vi "Main.vi"() -> ()   [LabVIEW 2014]
doc: "This Continuous Measurement sample project is based on the Queued Message Handler template.\n\nThe Event Handling Loop generates messages based on user interface actions.\n\nThe Message Handling Loop processes messages generated by the Event Handling Loop, or by other messages. There are also Acquisition and Logging message handling loop subVIs, and a chart updating loop."
uses:
  Settings/Settings.ctl
  Acquisition/Hardware Configuration.ctl
  Logging/Logging Configuration.ctl
  controls/UI Data.ctl
  controls/UI State.ctl
  support/Message Queue/Enqueue Message (Single).vi
  <vilib>/Utility/error.llb/Error Cluster From Error Code.vi
  <vilib>/ErrorRing/Error Ring.xnode
  Acquisition/Acquisition.lvlib
  Logging/Logging.lvlib
  Settings/Settings.lvlib
  support/User Event - Stop/User Event - Stop.lvlib
  support/Message Queue/Message Queue.lvlib
panel:
  out "Data":waveform(dbl)[](graph)
  in  "UserMetaData":T1 {"Amplifier Model" items=["Select a Model", "AM 1700", "BMA 200"]}
  in  "Settings":bool
  in  "Start":bool
  in  "Stop":bool
  out "Status":string
  in  "Exit":bool
  # "Direct-To-Disk Long Term EOD Recording Software (TDMS Output) (1.0)"
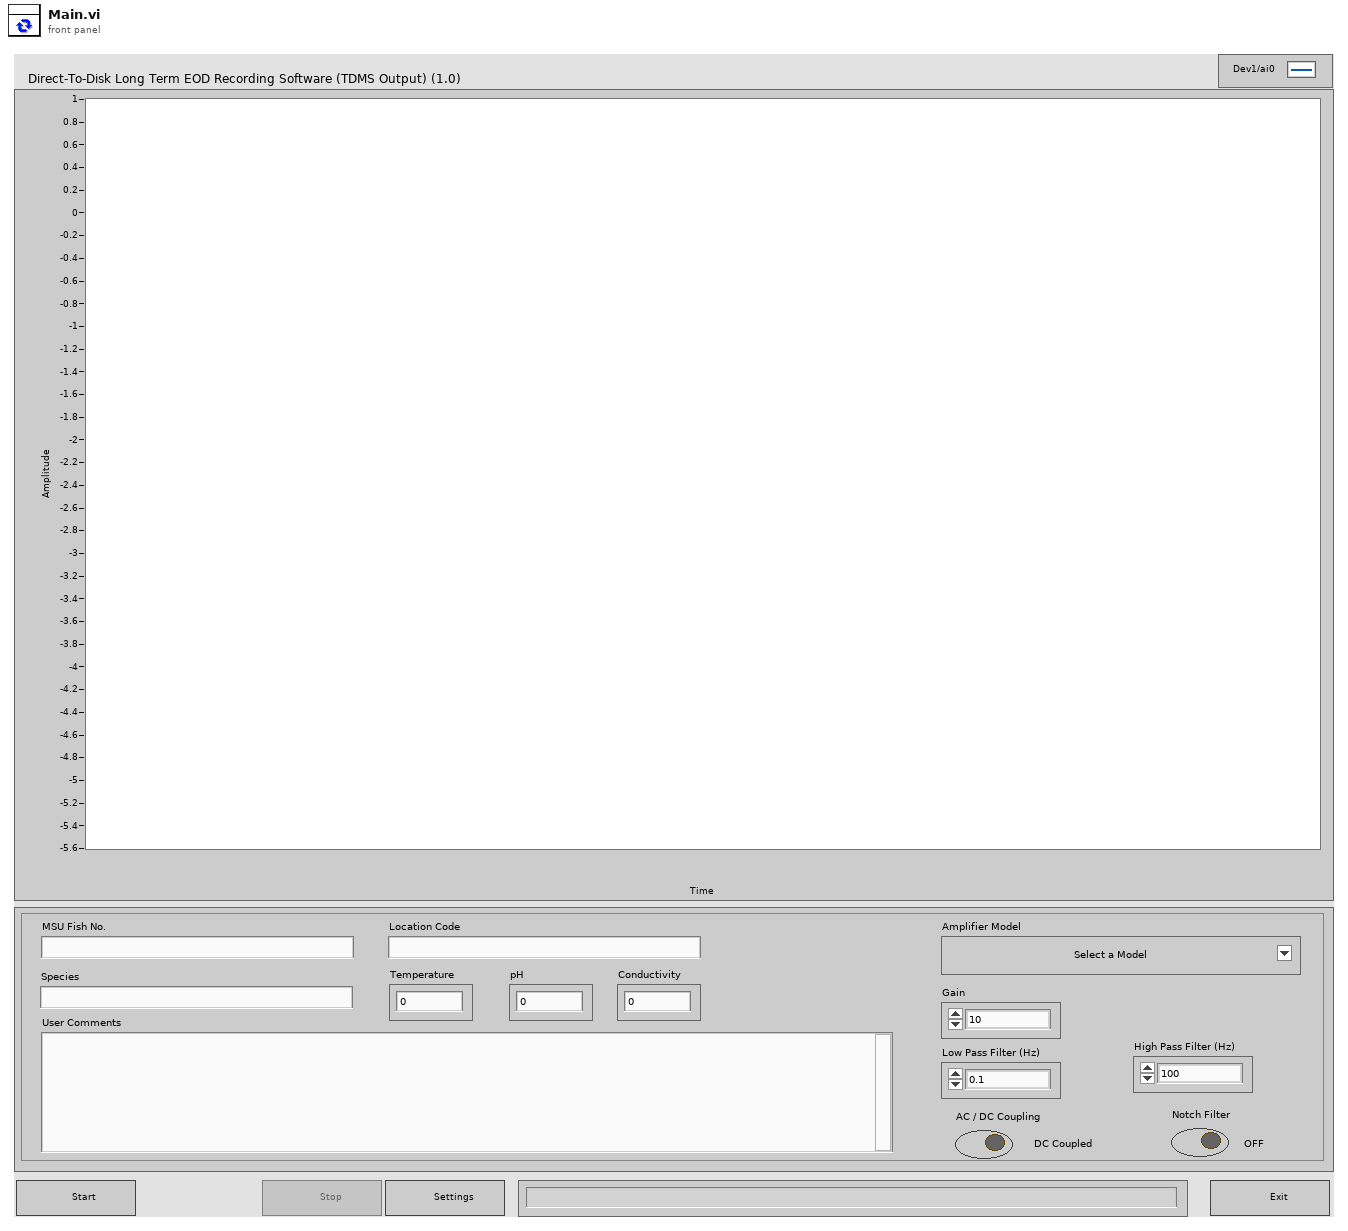
[diagram p1: front panel]
types:
  T1 = cluster{"MSU Fish No.":string, "Location Code":string, "Species":string, "Temperature":dbl, "pH":dbl, "Conductivity":dbl, "User Comments":string, "Amplifier Model":u16, "Gain":enum16{"10", "20", "50", "100", "200", "500", "1000", "2k", "5k", "10k", "20k", "50k"}, "Low Pass Filter (Hz)":enum16{"0.1", "1", "3", "10", "30", "100", "300"}, "High Pass Filter (Hz)":enum16{"100", "500", "1000", "3000", "5000", "10,000", "20,000", "30,000", "50,000"}, "AC / DC Coupling":bool, "Notch Filter":bool}
  T2 = typedef "UI State.ctl" = enum16{"Idle", "Acquiring and Logging", "Waiting for Exit", "Waiting for Exit (Acq Stopped)", "Waiting for Exit (Log Stopped)", "Waiting for Stop", "Waiting for Stop (Acq Stopped)", "Waiting for Stop (Log Stopped)"}
  T3 = typedef "UI Data.ctl" = cluster{"Start Ref":refnum<vi>, "Trigger Ref":refnum<vi>, "Stop Ref":refnum<vi>, "Settings Ref":refnum<vi>, "Status Ref":refnum<vi>, "Exit Ref":refnum<vi>, "Data Ref":refnum<vi>}
  T4 = typedef "Settings.lvlib/Settings.ctl" = cluster{"Hardware Configuration":T5, "Logging Configuration":T6}
  T5 = typedef "Acquisition.lvlib/Hardware Configuration.ctl" = cluster{"DAQmx Channel":tag, "Max Input":dbl, "Min Input":dbl, "Sample Rate":dbl, "DAQmx Task":refnum<k21>}
  T6 = typedef "Logging.lvlib/Logging Configuration.ctl" = cluster{"Log File Base Path":path, "TDMS File Reference":refnum<k34>, "Samples to Save":u32, "Trigger - Time":u32, "Trigger - Threshold":dbl, "Trigger - Channel":u32, "Enable Time Trigger":bool, "Enable Threshold Trigger":bool, "Always Log":bool}
  T7 = typedef "Message Queue.lvlib/All Message Queues.ctl" = cluster{"UI":refnum<queue>, "Acquisition":refnum<queue>, "Logging":refnum<queue>}
  T8 = enum8{"Enabled", "Disabled", "Disabled and Grayed Out"}
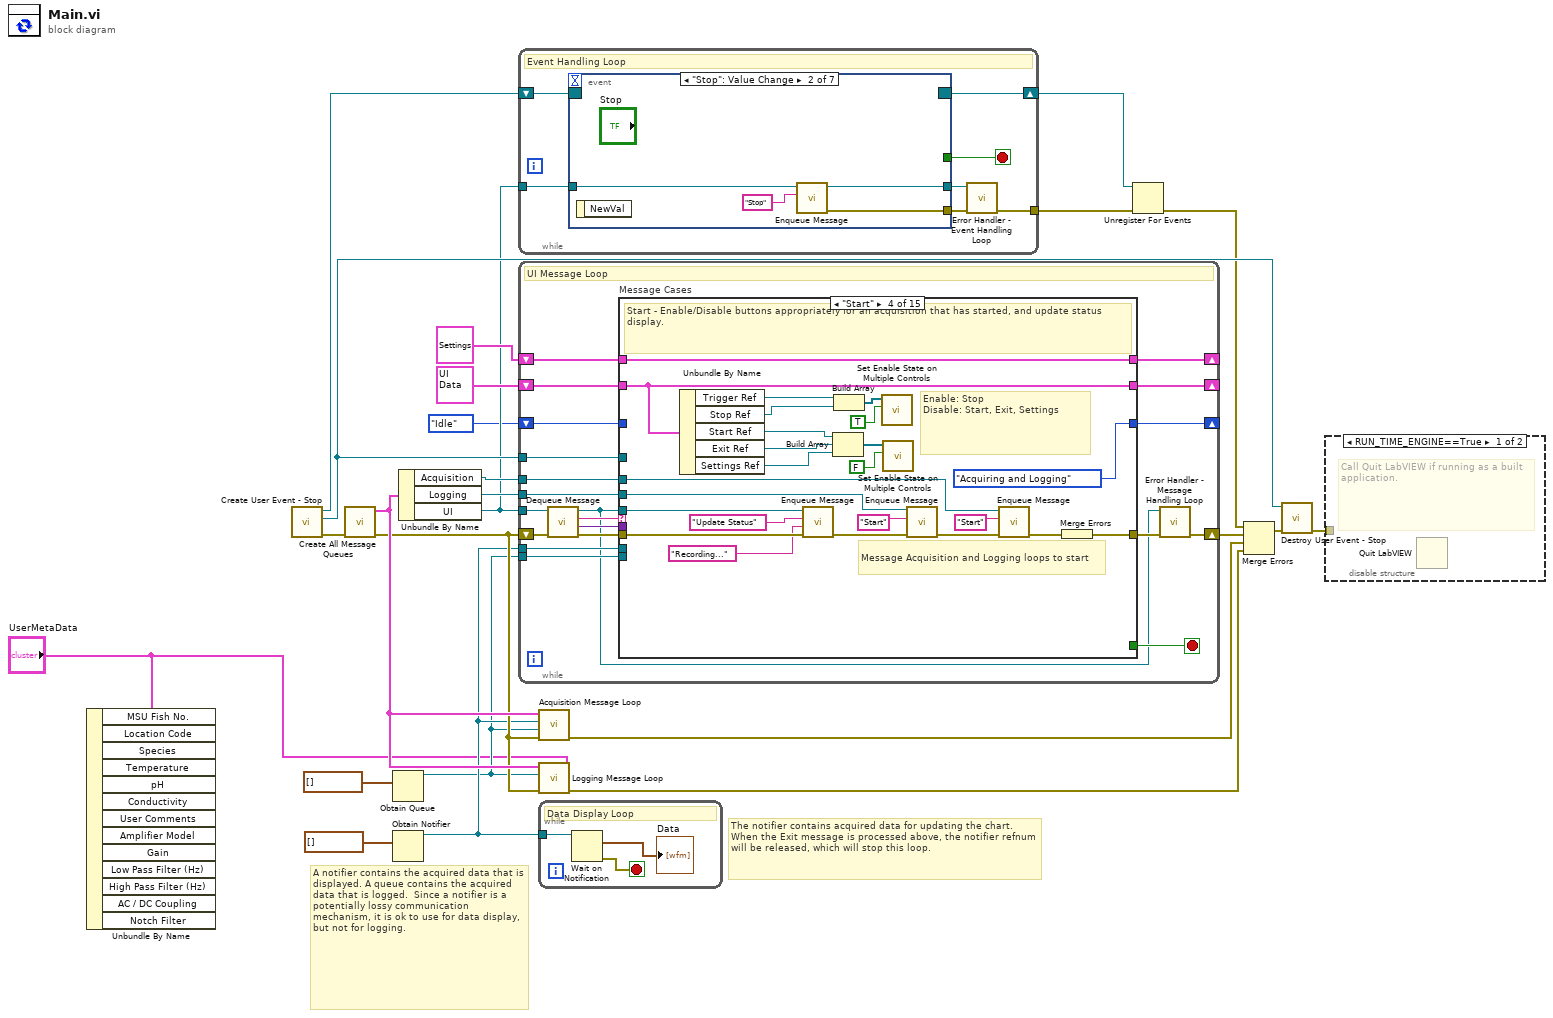
[diagram p0: block diagram]
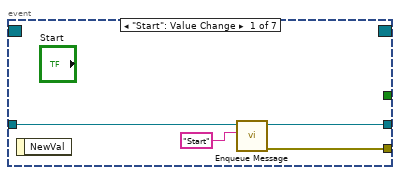
[diagram p3: hidden frame]
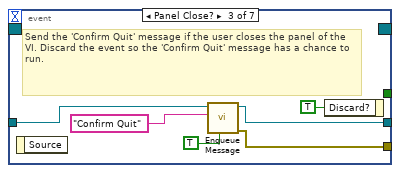
[diagram p4: hidden frame]
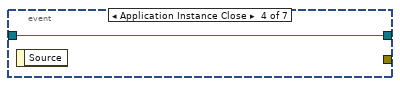
[diagram p5: hidden frame]
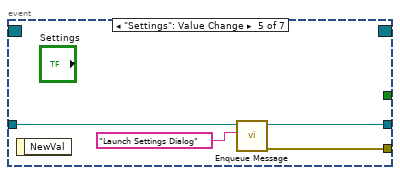
[diagram p6: hidden frame]
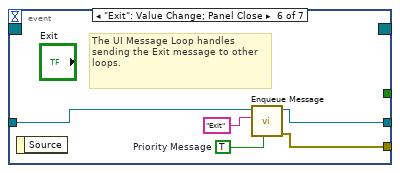
[diagram p7: hidden frame]
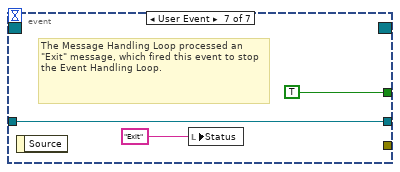
[diagram p8: hidden frame]
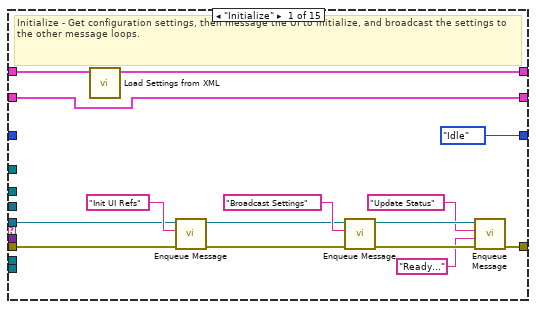
[diagram p9: hidden frame]
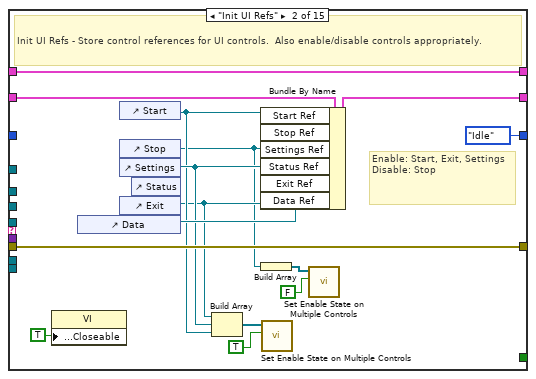
[diagram p10: hidden frame]
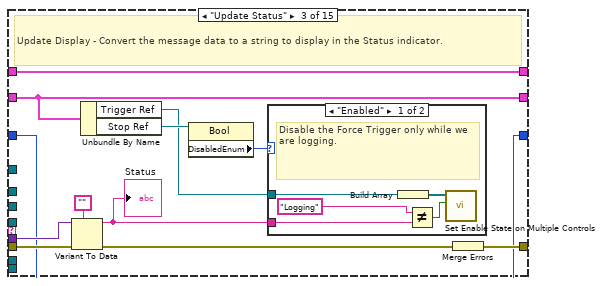
[diagram p11: hidden frame]
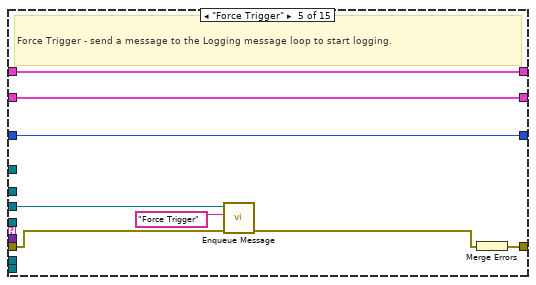
[diagram p13: hidden frame]
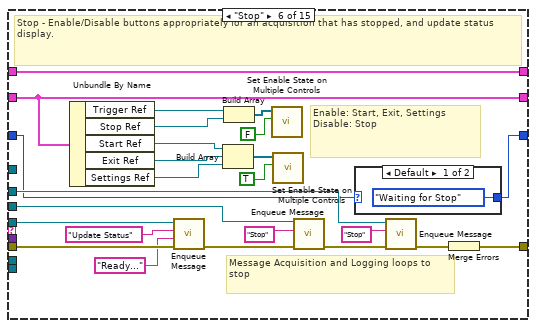
[diagram p14: hidden frame]
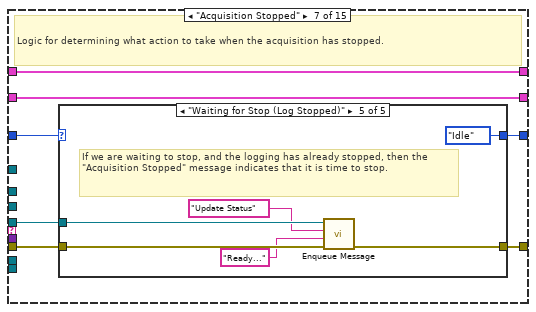
[diagram p16: hidden frame]
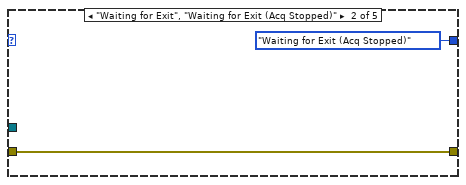
[diagram p18: hidden frame]
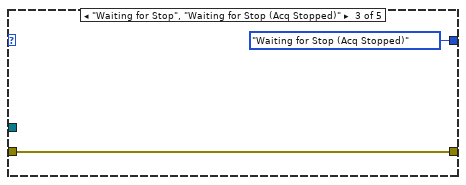
[diagram p19: hidden frame]
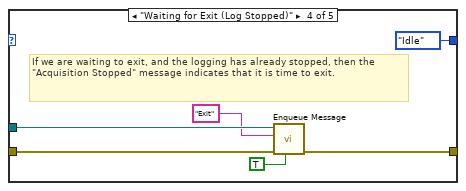
[diagram p20: hidden frame]
diagram:
  # "A notifier contains the acquired data that is displayed. A queue contains the acquired data that is logged.  Since a notifier is a potentially lossy communication mechanism, it is ok to use for data display, but not for logging."
  # "The notifier contains acquired data for updating the chart. When the Exit message is processed above, the notifier refnum will be released, which will stop this loop."
  n1 = Unbundle By Name("UserMetaData") -> ()  [unwired: 13 out]
  n2 = call "Create User Event - Stop.vi"() -> ("error out"=w18:errorcluster, "User Event - Stop"=w20:refnum<user-event>, "Stop Event Registration Refnum"=w21:refnum<event-registration>)  [unwired: 9 in]
  n3 = call "Create All Message Queues.vi"("error in (no error)"=w18) -> ("error out"=w15:errorcluster, "Message Queues out"=w17:T7)  [unwired: 9 in]
  n4 = Obtain Queue(element data type=waveform(dbl)[] []) -> (queue out=w4:refnum<queue>)  [unwired: 4 in, 2 out]
  n5 = Obtain Notifier(notification data type=waveform(dbl)[] []) -> (notifier out=w6:refnum<notifier>)  [unwired: 3 in, 2 out]
  n6 = Unbundle By Name(w17) -> ("Acquisition"=w10:refnum<queue>, "Logging"=w9:refnum<queue>, "UI"=w8:refnum<queue>)
  n7 = while {
    tunnel: w8 -> [w30]
    tunnel: [w25] -> w23
    shift-right: [w29] -> w12
    shift-left: w21 -> [w31]
    stop <- w28 stop-if-true
    # "Event Handling Loop"
    n8 = event shown="[1] \"Stop\": Value Change" {
      selector: w31 -> [_ _ _ _ _ _ _]
      dyn-events: [_ _ _ _ _ _ _] -> w29
      timeout: _ -> [_ _ _ _ _ _ _]
      tunnel: [_ _ _ _ _ _ TRUE ("Discard?")] -> w28
      tunnel: w30 -> [w33 w38 w45 w46 w48 w52 w56]
      tunnel: [w35 w37 w40 _ w50 w55 _] -> w26
      tunnel: [w32 w36 w41 w46 w47 w51 w56] -> w27
      event "Start": Value Change {
        n9 = event-data() -> ()  [unwired: 1 in, 1 out]
        n10 = call-poly "Enqueue Message.vi"("Message"="Start", "Message Queue"=w33) -> ("error out"=w35:errorcluster, "dup Message Queue"=w32:refnum<queue>)  [unwired: 8 in]
      }
      event "Stop": Value Change {
        n11 = event-data() -> ()  [unwired: 1 in, 1 out]
        n12 = call-poly "Enqueue Message.vi"("Message"="Stop", "Message Queue"=w38) -> ("error out"=w37:errorcluster, "dup Message Queue"=w36:refnum<queue>)  [unwired: 8 in]
      }
      event Panel Close? {
        # "Send the 'Confirm Quit' message if the user closes the panel of the VI. Discard the event so the 'Confirm Quit' message has a chance to run."
        n13 = event-data() -> ()  [unwired: 1 in, 1 out]
        n14 = call-poly "Enqueue Message.vi"("Priority Message? (F)"=TRUE, "Message"="Confirm Quit", "Message Queue"=w45) -> ("error out"=w40:errorcluster, "dup Message Queue"=w41:refnum<queue>)  [unwired: 7 in]
        n15 = event-data("Discard?"=TRUE) -> ()  [unwired: 1 in, 1 out]
      }
      event Application Instance Close {
        n16 = event-data() -> ()  [unwired: 1 in, 1 out]
      }
      event "Settings": Value Change {
        n17 = event-data() -> ()  [unwired: 1 in, 1 out]
        n18 = call-poly "Enqueue Message.vi"("Message"="Launch Settings Dialog", "Message Queue"=w48) -> ("error out"=w50:errorcluster, "dup Message Queue"=w47:refnum<queue>)  [unwired: 8 in]
      }
      event "Exit": Value Change; Panel Close {
        w53 = TRUE  # Priority Message
        # "The UI Message Loop handles sending the Exit message to other loops."
        n19 = event-data() -> ()  [unwired: 1 in, 1 out]
        n20 = call-poly "Enqueue Message.vi"("Priority Message? (F)"=w53, "Message"="Exit", "Message Queue"=w52) -> ("error out"=w55:errorcluster, "dup Message Queue"=w51:refnum<queue>)  [unwired: 7 in]
      }
      event User Event {
        # "The Message Handling Loop processed an \"Exit\" message, which fired this event to stop the Event Handling Loop."
        n21 = event-data() -> ()  [unwired: 1 in, 1 out]
        n22 = local write "Status"("Exit" ("Exit String")) -> ()
      }
    }
    n23 = call "Error Handler - Event Handling Loop.vi"("error in (no error)"=w26, "Message Queue"=w27) -> ("dup error in"=w25:errorcluster)  [unwired: 8 in, 1 out]
  }
  n24 = while {
    tunnel: w8 -> [w72]
    tunnel: w20 -> [w77]
    shift-right: [w62] -> w24
    shift-left: w15 -> [w76]
    shift-right: [w71] -> _
    shift-left: T4 {"Hardware Configuration"={"DAQmx Channel"="", "Max Input"=0.0, "Min Input"=0.0, "Sample Rate"=0.0, "DAQmx Task"=""}, "Logging Configuration"={"Log File Base Path"=path "", "TDMS File Reference"=refnum, "Samples to Save"=0, "Trigger - Time"=0, "Trigger - Threshold"=0.0, "Trigger - Channel"=0, "Enable Time Trigger"=FALSE, "Enable Threshold Trigger"=FALSE, "Always Log"=FALSE}} ("Settings") -> [w70]
    shift-right: [w68] -> _
    shift-left: T3 {"Start Ref"=refnum, "Trigger Ref"=refnum, "Stop Ref"=refnum, "Settings Ref"=refnum, "Status Ref"=refnum, "Exit Ref"=refnum, "Data Ref"=refnum} ("Measurement UI Controls") -> [w69]
    tunnel: w10 -> [w67]
    tunnel: w9 -> [w66]
    tunnel: w6 -> [w65]
    tunnel: w4 -> [w64]
    shift-right: [w59] -> _
    shift-left: UI_State."Idle" ("UI State") -> [w60]
    stop <- w78 stop-if-true
    # "UI Message Loop"
    n25 = call "Dequeue Message.vi"("error in (no error)"=w76, "Message Queue"=w72) -> ("error out"=w75:errorcluster, "Message Data"=w73:variant, "Message"=w74:string, "dup Message Queue"=w61:refnum<queue>)  [unwired: 6 in]
    n26 = case "Message Cases" shown="\"Start\"" w74 {
      selector: w74 -> [_ _ _ _ _ _ _ _ _ _ _ _ _ _ w328]
      tunnel: w61 -> [w83 _ _ w149 _ w182 w186 w211 _ w253 w268 w278 w311 _ _]
      tunnel: w75 -> [w82 w109 w120 w148 w155 w181 w188 w213 w241 w255 w272 w277 w319 w326 _]
      tunnel: [w89 w109 w121 w150 w158 w183 w187 w212 w247 w250 w263 w276 w320 w325 w329] -> w63
      tunnel: [_ _ _ _ _ _ _ _ _ _ _ _ TRUE _ _] -> w78
      tunnel: w73 -> [_ _ w119 _ _ _ _ _ _ _ w271 _ _ _ _]
      tunnel: w77 -> [_ _ _ _ _ _ _ _ _ _ _ _ w318 _ _]
      tunnel: [w92 w108 w116 w147 w157 w180 w192 w217 w245 w252 w274 w281 w316 w324 w331] -> w71
      tunnel: w70 -> [w93 w108 w116 w147 w157 w180 w192 w217 w245 w256 w274 w281 w316 w324 w331]
      tunnel: w69 -> [w85 w107 w115 w144 w156 w177 w191 w216 w239 w249 w273 w280 w314 w323 w330]
      tunnel: [w85 w106 w115 w144 w156 w177 w191 w216 w239 w249 w273 w280 w314 w323 w330] -> w68
      tunnel: w67 -> [_ _ _ w131 _ w164 _ _ w238 _ _ _ w313 _ _]
      tunnel: w66 -> [_ _ _ w134 w152 w167 _ _ w237 _ _ _ w312 _ _]
      tunnel: w65 -> [_ _ _ _ _ _ _ _ _ _ _ _ w310 _ _]
      tunnel: w64 -> [_ _ _ _ _ _ _ _ _ _ _ _ w306 _ _]
      tunnel: w60 -> [_ _ w110 _ w151 w160 w190 w215 w236 w248 w262 w279 _ w322 w327]
      tunnel: [UI_State."Idle" ("UI State") UI_State."Idle" ("UI State") w110 UI_State."Acquiring and Logging" ("UI State") w151 w159 w189 w214 w236 w248 w262 w275 UI_State."Idle" ("UI State") w322 w327] -> w59
      frame "Initialize" {
        # "Initialize - Get configuration settings, then message the UI to initialize, and broadcast the settings to the other message loops."
        n27 = call "Load Settings from XML.vi"("Settings in"=w93) -> ("Settings out"=w92:T4)  [unwired: 9 in, 1 out]
        n28 = call-poly "Enqueue Message.vi"("error in (no error)"=w82, "Message"="Init UI Refs", "Message Queue"=w83) -> ("error out"=w80:errorcluster, "dup Message Queue"=w81:refnum<queue>)  [unwired: 7 in]
        n29 = call-poly "Enqueue Message.vi"("error in (no error)"=w80, "Message"="Broadcast Settings", "Message Queue"=w81) -> ("error out"=w91:errorcluster, "dup Message Queue"=w90:refnum<queue>)  [unwired: 7 in]
        n30 = call-poly "Enqueue Message.vi"("error in (no error)"=w91, "Message Data"="Ready..." ("Ready..."), "Message"="Update Status", "Message Queue"=w90) -> ("error out"=w89:errorcluster)  [unwired: 6 in, 1 out]
      }
      frame "Init UI Refs" {
        # "Enable: Start, Exit, Settings\nDisable: Stop"
        # "Init UI Refs - Store control references for UI controls.  Also enable/disable controls appropriately."
        n31 = property class="VI"("Front Panel.Closeable"=TRUE ("Front Panel Window:Closeable")) -> ()  [unwired: 2 in, 2 out]
        n32 = control-ref of="Data"() -> (w102:refnum<vi>)
        n33 = control-ref of="Start"() -> (w101:refnum<vi>)
        n34 = control-ref of="Stop"() -> (w96:refnum<vi>)
        n35 = control-ref of="Settings"() -> (w98:refnum<vi>)
        n36 = control-ref of="Exit"() -> (w97:refnum<vi>)
        n37 = control-ref of="Status"() -> (w103:refnum<vi>)
        n38 = Build Array(w97, w98, w101) -> (w100:refnum<vi>[])
        n39 = Bundle By Name(cluster=w107, "Start Ref"=w101, "Stop Ref"=w96, "Settings Ref"=w98, "Status Ref"=w103, "Exit Ref"=w97, "Data Ref"=w102) -> (w106:T3)
        n40 = Build Array(w96) -> (w95:refnum<vi>[])
        n41 = call "Set Enable State on Multiple Controls.vi"("Enable?"=TRUE, "Controls"=w100) -> ()  [unwired: 10 in]
        n42 = call "Set Enable State on Multiple Controls.vi"("Enable?"=FALSE, "Controls"=w95) -> ()  [unwired: 10 in]
      }
      frame "Update Status" {
        # "Update Display - Convert the message data to a string to display in the Status indicator."
        n43 = Variant To Data(error in=w120, type="", Variant=w119) -> (data=w112:string, error out=w117:errorcluster)
        "Status" <- w112
        n44 = Unbundle By Name(w115) -> ("Trigger Ref"=w111:refnum<vi>, "Stop Ref"=w114:refnum<vi>)
        n45 = property class="Bool"(reference=w114) -> ("DisabledEnum"=w113:T8)  [unwired: 1 in, 2 out]
        n46 = case shown="\"Enabled\"" w113 {
          tunnel: w112 -> [w124 _]
          tunnel: w111 -> [w125 _]
          frame "Enabled" {
            # "Disable the Force Trigger only while we are logging."
            n47 = Build Array(w125) -> (w126:refnum<vi>[])
            n48 = Not Equal?(x="Logging" ("Logging"), y=w124) -> (x != y?=w122:bool)
            n49 = call "Set Enable State on Multiple Controls.vi"("Enable?"=w122, "Controls"=w126) -> ()  [unwired: 10 in]
          }
          frame "Disabled", Default {
          }
        }
        n50 = Merge Errors(w117) -> (w121:errorcluster)
      }
      frame "Start" {
        # "Message Acquisition and Logging loops to start"
        # "Enable: Stop\nDisable: Start, Exit, Settings"
        # "Start - Enable/Disable buttons appropriately for an acquisition that has started, and update status display."
        n51 = Unbundle By Name(w144) -> ("Trigger Ref"=w128:refnum<vi>, "Stop Ref"=w129:refnum<vi>, "Start Ref"=w139:refnum<vi>, "Exit Ref"=w138:refnum<vi>, "Settings Ref"=w137:refnum<vi>)
        n52 = call-poly "Enqueue Message.vi"("error in (no error)"=w148, "Message Data"="Recording..." ("Waiting for trigger"), "Message"="Update Status", "Message Queue"=w149) -> ("error out"=w136:errorcluster)  [unwired: 6 in, 1 out]
        n53 = Build Array(w139, w138, w137) -> (w142:refnum<vi>[])
        n54 = Build Array(w128, w129) -> (w141:refnum<vi>[])
        n55 = call "Set Enable State on Multiple Controls.vi"("Enable?"=TRUE, "Controls"=w141) -> ()  [unwired: 10 in]
        n56 = call "Set Enable State on Multiple Controls.vi"("Enable?"=FALSE, "Controls"=w142) -> ()  [unwired: 10 in]
        n57 = call-poly "Enqueue Message.vi"("error in (no error)"=w136, "Message"="Start", "Message Queue"=w134) -> ("error out"=w133:errorcluster)  [unwired: 7 in, 1 out]
        n58 = call-poly "Enqueue Message.vi"("error in (no error)"=w133, "Message"="Start", "Message Queue"=w131) -> ("error out"=w132:errorcluster)  [unwired: 7 in, 1 out]
        n59 = Merge Errors(w132) -> (w150:errorcluster)
      }
      frame "Force Trigger" {
        # "Force Trigger - send a message to the Logging message loop to start logging."
        n60 = call-poly "Enqueue Message.vi"("error in (no error)"=w155, "Message"="Force Trigger", "Message Queue"=w152) -> ("error out"=w154:errorcluster)  [unwired: 7 in, 1 out]
        n61 = Merge Errors(w154) -> (w158:errorcluster)
      }
      frame "Stop" {
        # "Message Acquisition and Logging loops to stop"
        # "Enable: Start, Exit, Settings\nDisable: Stop"
        # "Stop - Enable/Disable buttons appropriately for an acquisition that has stopped, and update status display."
        n62 = Unbundle By Name(w177) -> ("Trigger Ref"=w161:refnum<vi>, "Stop Ref"=w162:refnum<vi>, "Start Ref"=w172:refnum<vi>, "Exit Ref"=w171:refnum<vi>, "Settings Ref"=w170:refnum<vi>)
        n63 = call-poly "Enqueue Message.vi"("error in (no error)"=w181, "Message Data"="Ready..." ("Ready..."), "Message"="Update Status", "Message Queue"=w182) -> ("error out"=w169:errorcluster)  [unwired: 6 in, 1 out]
        n64 = Build Array(w172, w171, w170) -> (w175:refnum<vi>[])
        n65 = Build Array(w161, w162) -> (w174:refnum<vi>[])
        n66 = call "Set Enable State on Multiple Controls.vi"("Enable?"=FALSE, "Controls"=w174) -> ()  [unwired: 10 in]
        n67 = call "Set Enable State on Multiple Controls.vi"("Enable?"=TRUE, "Controls"=w175) -> ()  [unwired: 10 in]
        n68 = call-poly "Enqueue Message.vi"("error in (no error)"=w169, "Message"="Stop", "Message Queue"=w167) -> ("error out"=w166:errorcluster)  [unwired: 7 in, 1 out]
        n69 = case shown="Default" w160 {
          selector: w160 -> [_ w185]
          tunnel: [UI_State."Waiting for Stop" ("UI State") w185] -> w159
          frame Default {
          }
          frame "Waiting for Exit" {
          }
        }
        n70 = call-poly "Enqueue Message.vi"("error in (no error)"=w166, "Message"="Stop", "Message Queue"=w164) -> ("error out"=w165:errorcluster)  [unwired: 7 in, 1 out]
        n71 = Merge Errors(w165) -> (w183:errorcluster)
      }
      frame "Acquisition Stopped" {
        # "Logic for determining what action to take when the acquisition has stopped."
        n72 = case shown="\"Waiting for Stop (Log Stopped)\"" w190 {
          selector: w190 -> [w194 _ _ _ _]
          tunnel: [w194 UI_State."Waiting for Exit (Acq Stopped)" ("UI State") UI_State."Waiting for Stop (Acq Stopped)" ("UI State") UI_State."Idle" ("UI State") UI_State."Idle" ("UI State")] -> w189
          tunnel: w188 -> [w193 w195 w197 w203 w209]
          tunnel: [w193 w195 w197 w202 w208] -> w187
          tunnel: w186 -> [_ _ _ w201 w207]
          frame Default {
          }
          frame "Waiting for Exit", "Waiting for Exit (Acq Stopped)" {
          }
          frame "Waiting for Stop", "Waiting for Stop (Acq Stopped)" {
          }
          frame "Waiting for Exit (Log Stopped)" {
            # "If we are waiting to exit, and the logging has already stopped, then the \"Acquisition Stopped\" message indicates that it is time to exit."
            n73 = call-poly "Enqueue Message.vi"("Priority Message? (F)"=TRUE, "error in (no error)"=w203, "Message"="Exit", "Message Queue"=w201) -> ("error out"=w202:errorcluster)  [unwired: 6 in, 1 out]
          }
          frame "Waiting for Stop (Log Stopped)" {
            # "If we are waiting to stop, and the logging has already stopped, then the \"Acquisition Stopped\" message indicates that it is time to stop."
            n74 = call-poly "Enqueue Message.vi"("error in (no error)"=w209, "Message Data"="Ready..." ("Message"), "Message"="Update Status", "Message Queue"=w207) -> ("error out"=w208:errorcluster)  [unwired: 6 in, 1 out]
          }
        }
      }
      frame "Logging Stopped" {
        # "Logic for determining what action to take when the logging has stopped."
        n75 = case shown="\"Waiting for Stop (Acq Stopped)\"" w215 {
          selector: w215 -> [w219 _ _ _ _]
          tunnel: [w219 UI_State."Waiting for Exit (Log Stopped)" ("UI State") UI_State."Waiting for Stop (Log Stopped)" ("UI State") UI_State."Idle" ("UI State") UI_State."Idle" ("UI State")] -> w214
          tunnel: w213 -> [w218 w220 w222 w228 w234]
          tunnel: [w218 w220 w222 w227 w233] -> w212
          tunnel: w211 -> [_ _ _ w226 w232]
          frame Default {
          }
          frame "Waiting for Exit", "Waiting for Exit (Log Stopped)" {
          }
          frame "Waiting for Stop", "Waiting for Stop (Log Stopped)" {
          }
          frame "Waiting for Exit (Acq Stopped)" {
            # "If we are waiting to exit, and the acquisition has already stopped, then the \"Logging Stopped\" message indicates that it is time to exit."
            n76 = call-poly "Enqueue Message.vi"("Priority Message? (F)"=TRUE, "error in (no error)"=w228, "Message"="Exit", "Message Queue"=w226) -> ("error out"=w227:errorcluster)  [unwired: 6 in, 1 out]
          }
          frame "Waiting for Stop (Acq Stopped)" {
            # "If we are waiting to stop, and the acquisition has already stopped, then the \"Logging Stopped\" message indicates that it is time to stop."
            n77 = call-poly "Enqueue Message.vi"("error in (no error)"=w234, "Message Data"="Ready..." ("Message"), "Message"="Update Status", "Message Queue"=w232) -> ("error out"=w233:errorcluster)  [unwired: 6 in, 1 out]
          }
        }
      }
      frame "Broadcast settings" {
        w240 = "Update Settings" ("Message")
        # "Send the 'Update Settings' message to the Logging and Acquisition message loops."
        n78 = Unbundle By Name(w245) -> ("Hardware Configuration"=w244:T5, "Logging Configuration"=w243:T6)
        n79 = call-poly "Enqueue Message.vi"("Message Data"=w244, "Message"=w240, "Message Queue"=w238) -> ("error out"=w246:errorcluster)  [unwired: 7 in, 1 out]
        n80 = call-poly "Enqueue Message.vi"("error in (no error)"=w246, "Message Data"=w243, "Message"=w240, "Message Queue"=w237) -> ("error out"=w242:errorcluster)  [unwired: 6 in, 1 out]
        n81 = Merge Errors(w242, w241) -> (w247:errorcluster)
      }
      frame "Launch Settings Dialog" {
        # "Launch the Settings Dialog when the user clicks the 'Settings' button."
        n82 = call "Settings Dialog.vi"("error in (no error)"=w255, "Settings in"=w256) -> ("error out"=w251:errorcluster, "Cancelled?"=w254:bool, "Settings out"=w252:T4)  [unwired: 6 in, 1 out]
        n83 = case shown="False" w254 {
          tunnel: w253 -> [w260 _]
          tunnel: w251 -> [w259 w261]
          tunnel: [w258 w261] -> w250
          frame False {
            n84 = call-poly "Enqueue Message.vi"("error in (no error)"=w259, "Message"="Broadcast Settings", "Message Queue"=w260) -> ("error out"=w258:errorcluster)  [unwired: 7 in, 1 out]
          }
          frame True {
          }
        }
      }
      frame "Error" {
        # "Error - Check the error message data and respond accordingly. This message is sent by the \"Error Handler\" VIs at the end of each loop in this application."
        n85 = Variant To Data(error in=w272, type=errorcluster {"status"=FALSE, "code"=0, "source"=""} ("error out"), Variant=w271) -> (data=w269:errorcluster, error out=w265:errorcluster)
        n86 = call <vilib>:"Simple Error Handler.vi"("error in (no error)"=w269) -> ()  [unwired: 4 in, 5 out]
        n87 = call-poly "Enqueue Message.vi"("Priority Message? (F)"=TRUE, "Message"="Exit", "Message Queue"=w268) -> ("error out"=w264:errorcluster)  [unwired: 7 in, 1 out]
        n88 = Merge Errors(w264, w265) -> (w263:errorcluster)
      }
      frame "Confirm Quit" {
        # "Confirm Quit - Message that can confirm whether or not the user wants to exit the application."
        n89 = case shown="\"Acquiring and Logging\"" w279 {
          tunnel: w278 -> [w286 w292]
          tunnel: w277 -> [w285 w290]
          tunnel: [w282 w289] -> w276
          tunnel: [UI_State."Idle" ("UI State") w288] -> w275
          frame Default {
            # "If 'Confirm Quit' comes in while the system is idle, there is no need for a confirmation message."
            n90 = call-poly "Enqueue Message.vi"("Priority Message? (F)"=TRUE, "error in (no error)"=w285, "Message"="Exit", "Message Queue"=w286) -> ("error out"=w282:errorcluster)  [unwired: 6 in, 1 out]
          }
          frame "Acquiring and Logging" {
            n91 = Two Button Dialog(message="Are you sure you want to quit while the acquisition is running?" ("Confirm Quit Message"), 1:"No" ("No"), 2:"Yes" ("Yes")) -> (T button?=w291:bool)
            n92 = case shown="True" w291 {
              tunnel: w292 -> [_ w302]
              tunnel: w290 -> [w296 w301]
              tunnel: [w296 w300] -> w289
              tunnel: [UI_State."Acquiring and Logging" ("UI State") UI_State."Waiting for Exit" ("UI State")] -> w288
              frame False {
                # "User did not want to quit."
              }
              frame True {
                n93 = call-poly "Enqueue Message.vi"("error in (no error)"=w301, "Message"="Stop", "Message Queue"=w302) -> ("error out"=w300:errorcluster)  [unwired: 7 in, 1 out]
              }
            }
          }
        }
      }
      frame "Exit" {
        w315 = "Exit" ("Message")
        # "Don't check the error outs. The acquisition and logging queues may have already been released."
        # "Close references owned by the Main VI."
        # "Stop the VI"
        # "Exit - Fire the User Event to stop the Event Handling Loop.  Also send Exit messages to the Acquisition and Logging loops."
        n94 = Release Queue(queue=w311, error in (no error)=w319) -> (error out=w309:errorcluster)  [unwired: 1 in, 2 out]
        n95 = call "Fire User Event - Stop.vi"("User Event - Stop"=w318) -> ("error out"=w317:errorcluster)  [unwired: 10 in]
        n96 = Release Notifier(notifier=w310, error in (no error)=w309) -> (error out=w308:errorcluster)  [unwired: 1 in, 2 out]
        n97 = Release Queue(queue=w306, error in (no error)=w308) -> (error out=w307:errorcluster)  [unwired: 1 in, 2 out]
        n98 = call-poly "Enqueue Message.vi"("Priority Message? (F)"=TRUE, "Message"=w315, "Message Queue"=w313) -> ()  [unwired: 7 in, 2 out]
        n99 = call-poly "Enqueue Message.vi"("Priority Message? (F)"=TRUE, "Message"=w315, "Message Queue"=w312) -> ()  [unwired: 7 in, 2 out]
        n100 = Merge Errors(w317, w307) -> (w320:errorcluster)
      }
      frame "---Copy This Frame---" {
        # "Duplicate this frame when creating new messages.  Change this comment in the duplicated frame to describe this message."
        n101 = Merge Errors(w326) -> (w325:errorcluster)
      }
      frame Default {
        # "'Default' case only runs if there is a message that isn't defined in any of the other cases.  Output a programming error."
        n102 = xnode "Error Ring"("parameter 0"=w328) -> ("error out"=w329:errorcluster)
      }
    }
    n103 = call "Error Handler - Message Handling Loop.vi"("error in (no error)"=w63, "Message Queue"=w61) -> ("dup error in"=w62:errorcluster)  [unwired: 8 in, 1 out]
  }
  n104 = call "Acquisition Message Loop.vi"("error in (no error)"=w15, "Data Queue"=w4, "Data Notifier"=w6, "Message Queues"=w17) -> ("error out"=w19:errorcluster)  [unwired: 7 in]
  n105 = call "Logging Message Loop.vi"("UserMetaData"="UserMetaData", "error in (no error)"=w15, "Data Queue"=w4, "Message Queues"=w17) -> ("error out"=w16:errorcluster)  [unwired: 7 in]
  n106 = while "Data Display Loop" {
    tunnel: w6 -> [w341]
    stop <- w339 stop-if-true
    # "Data Display Loop"
    n107 = Wait on Notification(notifier=w341) -> (notification=→"Data":waveform(dbl)[], error out=w339:errorcluster)  [unwired: 3 in, 2 out]
  }
  n108 = Unregister For Events(event registration refnum=w12, error in=w23) -> (error out=w13:errorcluster)
  n109 = Merge Errors(w13, w24, w19, w16) -> (w22:errorcluster)
  n110 = call "Destroy User Event - Stop.vi"("error in (no error)"=w22, "User Event - Stop"=w20) -> ("error out"=w3:errorcluster)  [unwired: 9 in]
  n111 = disable-structure shown="RUN_TIME_ENGINE==True" {
    disable-tunnel: w3 -> [_ _]
    frame condition #0 {
      # "Call Quit LabVIEW if running as a built application."
      n112 = Quit LabVIEW() -> ()  [unwired: 1 in]
    }
    frame condition #1 (active) {
    }
  }
